vi "Get_No_Top_Level_Message.vi"(11 "Build in":refnum<class "AB_SourceDistribution.lvclass">) -> (2 "No top level VI":string, 3 "Build out":refnum<class "AB_SourceDistribution.lvclass">)   [LabVIEW 2020, in "AB_SourceDistribution.lvclass"]
uses:
  <vilib>/AppBuilder/AB_Classes/SourceDistribution/AB_SourceDistribution.lvclass
  <resource>/Framework/Providers/Common/provcom_StringGlobals.vi
  <vilib>/AppBuilder/AB_Classes/SourceDistribution/AB_SourceDistribution.lvclass/AB_SourceDistribution.ctl
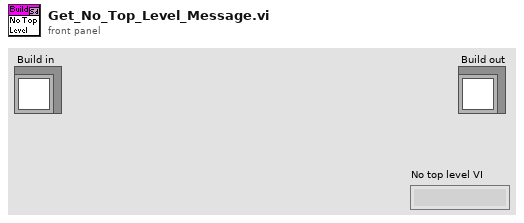
[diagram p1: front panel]
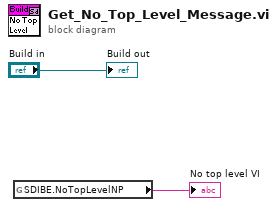
[diagram p0: block diagram]
diagram:
  n1 = global read "provcom_StringGlobals.vi" "SDIBE.NoTopLevelNP"() -> (→"No top level VI":string)
  "Build out" <- "Build in"
